vi "MOTOR Action-Status Move Single.vi"(8 "error in (no error)":errorcluster, 10 "Message Data":variant, 11 "Data Cluster in":T1={"Tango HW"={"VISA resource"="", "Baud Rate (115200)"=2, "lAnInterfaceType"=0, "bAShowProt"=15}, "Writer Queue"=refnum, "Status"=FALSE, "Abs Position"=[], "Axis Velocity"={"dX"=0.0, "dY"=0.0, "dZ"=0.0, "dA"=0.0}, "acceleration "=0.0, "Z direction"=enum."Up", "Position Mode"="", "plLSID"=0}) -> (0 "error out":errorcluster, 3 "Data Cluster out":T1={"Tango HW"={"VISA resource"="", "Baud Rate (115200)"=2, "lAnInterfaceType"=0, "bAShowProt"=15}, "Writer Queue"=refnum, "Status"=FALSE, "Abs Position"=[], "Axis Velocity"={"dX"=0.0, "dY"=0.0, "dZ"=0.0, "dA"=0.0}, "acceleration "=0.0, "Z direction"=enum."Up", "Position Mode"="", "plLSID"=0})   [LabVIEW 2020, in "MOTOR.lvlib"]
uses:
  MOTOR.lvlib
  PS Hardware Configuration.ctl
  support/Message Queue/Message Cluster.ctl
  support/HW Message Cluster.ctl
  support/PCT FGV CMD.ctl
  support/Message Queue/Enqueue Message (Single).vi
  support/Message Queue/Message Queue.lvlib
  <instrlib>/Tango_DLL/Tango_DLL.lvlib
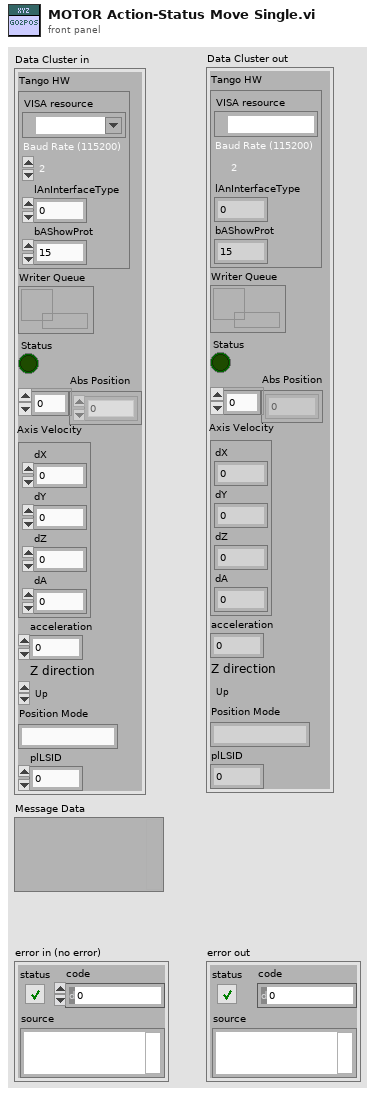
[diagram p1: front panel]
types:
  T1 = typedef "MOTOR.lvlib/PS Hardware Configuration.ctl" = cluster{"Tango HW":cluster{"VISA resource":refnum<visa-resource-name>, "Baud Rate (115200)":i32, "lAnInterfaceType":i32, "bAShowProt":i32}, "Writer Queue":refnum<queue>, "Status":bool, "Abs Position":i32[], "Axis Velocity":cluster{"dX":dbl, "dY":dbl, "dZ":dbl, "dA":dbl}, "acceleration ":dbl, "Z direction":enum16{"Up", "Down"}, "Position Mode":string, "plLSID":i32}
  T2 = typedef "PCT FGV CMD.ctl" = enum16{"INIT", "GET", "SET"}
  T3 = cluster{"Axis":enum16{"X", "Y", "Z", "A"}, "dValue":dbl}
  T4 = typedef "Message Queue.lvlib/HW Message Cluster.ctl" = cluster{"Writer Queue":refnum<queue>, "Writer Data":T5}
  T5 = typedef "Message Queue.lvlib/Message Cluster.ctl" = cluster{"Message":string, "Message Data":variant}
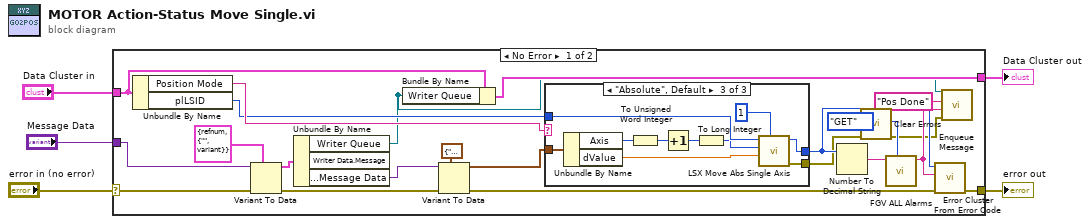
[diagram p0: block diagram]
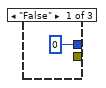
[diagram p2: hidden frame]
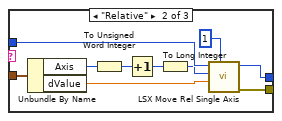
[diagram p3: hidden frame]
diagram:
  n1 = case shown="No Error" "error in (no error)" {
    selector: "error in (no error)" -> [w22 w49]
    tunnel: "Message Data" -> [w21 _]
    tunnel: [w20 w50] -> w4
    tunnel: "Data Cluster in" -> [w13 w50]
    tunnel: [w17 w49] -> w2
    frame No Error {
      n2 = Unbundle By Name(w13) -> ("Position Mode"=w12:string, "plLSID"=w11:i32)
      n3 = Variant To Data(error in=w22, type=T4 {"Writer Queue"=refnum, "Writer Data"={"Message"="", "Message Data"=variant}}, Variant=w21) -> (data=w23:T4, error out=w25:errorcluster)
      n4 = Unbundle By Name(w23) -> ("Writer Queue"=w10:refnum<queue>, "Writer Data.Message Data"=w24:variant)  [unwired: 1 out]
      n5 = Bundle By Name(cluster=w13, "Writer Queue"=w10) -> (w20:T1)
      n6 = Variant To Data(error in=w25, type=T3 {"Axis"=enum."X", "dValue"=0.0}, Variant=w24) -> (data=w18:T3, error out=w27:errorcluster)
      n7 = case shown="\"Absolute\", Default" w12 {
        tunnel: w18 -> [_ w38 w48]
        tunnel: [0 ("function return") w30 w40] -> w14
        tunnel: w11 -> [_ w34 w44]
        tunnel: [_ w29 w39] -> w7
        frame "False" {
        }
        frame "Relative" {
          n8 = Unbundle By Name(w38) -> ("Axis"=w37:enum16{"X", "Y", "Z", "A"}, "dValue"=w33:dbl)
          n9 = To Unsigned Word Integer(number=w37) -> (unsigned 16bit integer=w36:u16)
          n10 = Increment(x=w36) -> (x+1=w35:u16)
          n11 = To Long Integer(number=w35) -> (32bit integer=w32:i32)
          n12 = call <instrlib>:"LSX Move Rel Single Axis.vi"("bWait"=1, "dValue"=w33, "lAxis"=w32, "lLSID"=w34) -> ("error out"=w29:errorcluster, "function return"=w30:i32)  [unwired: 6 in]
        }
        frame "Absolute", Default {
          n13 = Unbundle By Name(w48) -> ("Axis"=w47:enum16{"X", "Y", "Z", "A"}, "dValue"=w42:dbl)
          n14 = To Unsigned Word Integer(number=w47) -> (unsigned 16bit integer=w46:u16)
          n15 = Increment(x=w46) -> (x+1=w45:u16)
          n16 = To Long Integer(number=w45) -> (32bit integer=w43:i32)
          n17 = call <instrlib>:"LSX Move Abs Single Axis.vi"("bWait"=1, "dValue"=w42, "lAxis"=w43, "lLSID"=w44) -> ("error out"=w39:errorcluster, "function return"=w40:i32)  [unwired: 6 in]
        }
      }
      n18 = Number To Decimal String(number=w14) -> (decimal integer string=w15:string)  [unwired: 1 in]
      n19 = call <vilib>:"Clear Errors.vi"("error in (no error)"=w7) -> ("error out"=w6:errorcluster)  [unwired: 5 in, 1 out]
      n20 = call "FGV ALL Alarms.vi"("CMD"=PCT_FGV_CMD."GET", "name"=w15) -> ("Alarm MSG out"=w8:string)  [unwired: 8 in, 1 out]
      n21 = call <vilib>:"Error Cluster From Error Code.vi"("error in (no error)"=w27, "error message (\"\")"=w8, "error code (0)"=w14) -> ("error out"=w17:errorcluster)  [unwired: 6 in]
      n22 = call-poly "Enqueue Message.vi"("error in (no error)"=w6, "Message Data"=w8, "Message"="Pos Done", "Message Queue"=w10) -> ()  [unwired: 6 in, 2 out]
    }
    frame Error {
    }
  }
  "Data Cluster out" <- w4
  "error out" <- w2
